vi "Waveform Acquisition - Process (4xI16).vi"(2 "Waveform Acquisition Resources":T1) -> ()   [LabVIEW 2018, in "Streaming FPGA.lvlib"]
doc: "Waveform Acquisition processing VI.\n\nConnect the <B>Waveform Acquisition Resources</B> input of this VI to the output of the <B>Waveform Acquisition - Create Resources.vi</B>."
uses:
  Streaming FPGA.lvlib
  Waveform Acquisition Resources (4xI16).ctl
  Target-Scoped FIFO (4xI16) Resource.ctl
  <vilib>/Platform/TimedLoop/XDataNode/timing_clust.ctl
  <vilib>/Platform/TimedLoop/XDataNode/nitl_modes.ctl
  <vilib>/Platform/TimedLoop/XDataNode/wakeup.ctl
  Data Storage - DRAM FIFO Priority.ctl
  <vilib>/rvi/Emulation/niFpgaSctlEmulationGetInTimedLoop.vi
  <vilib>/rvi/Emulation/niFpgaEmulationReportErrorSimple.vi
  <vilib>/rvi/Emulation/niFpgaGetClockAttributes.vi
  <vilib>/rvi/Emulation/niFpgaCriticalErrorInLSC.vi
  <vilib>/rvi/DataTransferAndStorage/Container/Common/niFpgaContainerExecOnDevCompGetState.vi
  <vilib>/rvi/Emulation/niFpgaEmulationIsFPGAContextNoSignature.vi
  <vilib>/rvi/DataTransferAndStorage/Container/Common/niFpgaContainerGetUniqueNameForEmu.vi
  <vilib>/rvi/Memory/Memory_Emulation/niFpgaMemoryEmulationCacheClearOnFirstRun.vi
  <vilib>/rvi/Memory/Memory_Emulation/nirvimemoryEmulationManagerCache_MakeExclusive.vi
  <vilib>/rvi/Memory/Memory_Emulation/niFpgaMemoryEmulationValidateCache.vi
  <vilib>/rvi/Memory/Memory_Emulation/nirvimemoryEmulationManagerCache_InsertValue.vi
  <vilib>/Utility/error.llb/Clear Errors.vi
  <vilib>/rvi/Memory/Memory_Emulation/nirvimemoryEmulationManagerCache_ReleaseExclusive.vi
  <vilib>/rvi/Memory/Memory_Emulation/nirvimemoryEmulationManagerCache_GetValue.vi
  <vilib>/rvi/Memory/Memory_Emulation/nirvimemoryEmulationManagerCache_SetValue.vi
  <vilib>/rvi/Emulation/niFpgaProcessEmulError.vi
  <instrlib>/_niInstr/Basic Elements/v1/FPGA/Private/Count Up U32.vi
  <vilib>/rvi/errors/niFpgaSetErrorForExecOnDevCompSimple.vi
  <vilib>/rvi/eio/common/nirviEmuReportErrorAndStop.vi
  <vilib>/rvi/interface/RandomDataEmulation/nirviRandomDataAcquireLock.vi
  <vilib>/rvi/interface/RandomDataEmulation/nirviRandomDataQueueStore.vi
  <vilib>/rvi/interface/RandomDataEmulation/nirviRandomDataReleaseLock.vi
  <vilib>/rvi/interface/RandomDataEmulation/nirviFPGAContextMergeError.vi
  <vilib>/rvi/interface/RandomDataEmulation/nirviRandomDataCheckExitLoopConditions.vi
  <vilib>/express/rvi/timingcommon/nirviCommon.vi
  <vilib>/rvi/interface/RandomDataEmulation/niFpgaRandomDataHandleErrors.vi
  <vilib>/platform/TimedLoop/XDataNode/XDataNode.xnode
  <vilib>/rvi/DataTransferAndStorage/Container/XNode/niFpgaContainer.xnode
  <vilib>/rvi/DataTransferAndStorage/Register/Emulation/niFpgaRegisterEmulationRefIn.vi
  <vilib>/rvi/FIFO/Fifo_Resource/niFpgaFifoEmulationRefInMultiElement.vi
  <vilib>/Platform/TimedLoop/XDataNode/XDNodeRunTimeDep.lvlib
  <instrlib>/_niInstr/Basic Elements/v1/FPGA/niInstr Basic Elements v1 FPGA.lvlib
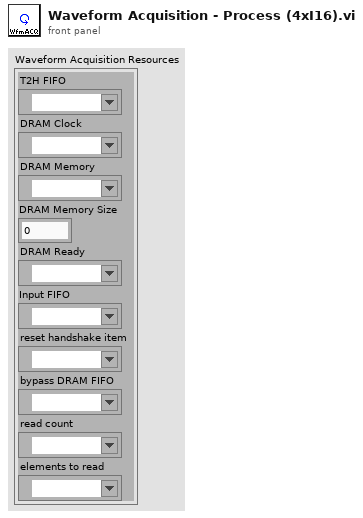
[diagram p1: front panel]
types:
  T1 = typedef "Streaming FPGA.lvlib/Waveform Acquisition Resources (4xI16).ctl" = cluster{"T2H FIFO":refnum<k21>, "DRAM Clock":refnum<k21>, "DRAM Memory":refnum<k21>, "DRAM Memory Size":u32, "DRAM Ready":refnum<k21>, "Input FIFO":T2, "reset handshake item":refnum<k21>, "bypass DRAM FIFO":refnum<k21>, "read count":refnum<k21>, "elements to read":refnum<k21>}
  T2 = typedef "Streaming FPGA.lvlib/Target-Scoped FIFO (4xI16) Resource.ctl" = refnum<k21>
  T3 = typedef "XDNodeRunTimeDep.lvlib/timing_clust.ctl" = cluster{"Expected End [f-1]":u64, "Actual End [f-1]":u64, "Finished Late? [f-1]":bool, "Expected End [i-1]":u64, "Actual End [i-1]":u64, "Finished Late? [i-1]":bool, "Expected Start [i]":u64, "Actual Start [i]":u64, "Expected Start [f]":u64, "Actual Start [f]":u64, "Source Name":string, "Structure Name":string, "Period":i64, "Deadline":i64, "Offset":i64, "Start":i64, "Priority":i32, "Timeout":i32, "Mode":T4, "Wakeup Reason":T5, "Error":errorcluster, "Source Type":string, "Secondary Source Type":string, "Global End Time":u64, "Global Start Time":u64, "Frame Duration":u64, "Iteration Duration":u64, "Assigned CPU":i32, "I/O Scan Engine Mode":u32}
  T4 = typedef "XDNodeRunTimeDep.lvlib/nitl_modes.ctl" = enum32{"No Change", "Process missed periods, maintain original phase", "Discard missed periods, maintain original phase", "Process missed periods, ignore original phase", "Discard missed periods, ignore original phase"}
  T5 = typedef "XDNodeRunTimeDep.lvlib/wakeup.ctl" = enum32{"Normal", "Aborted", "Asynchronous wakeup", "Timing source error", "Timed loop error", "Timeout"}
  T6 = typedef "Streaming FPGA.lvlib/Data Storage - DRAM FIFO Priority.ctl" = enum16{"balanced", "favor writes", "favor reads"}
  T7 = typedef "Streaming FPGA.lvlib/Data Type (4xI16).ctl" = i16[]
  T8 = typedef "Streaming FPGA.lvlib/Data Type (16xI16).ctl" = i16[]
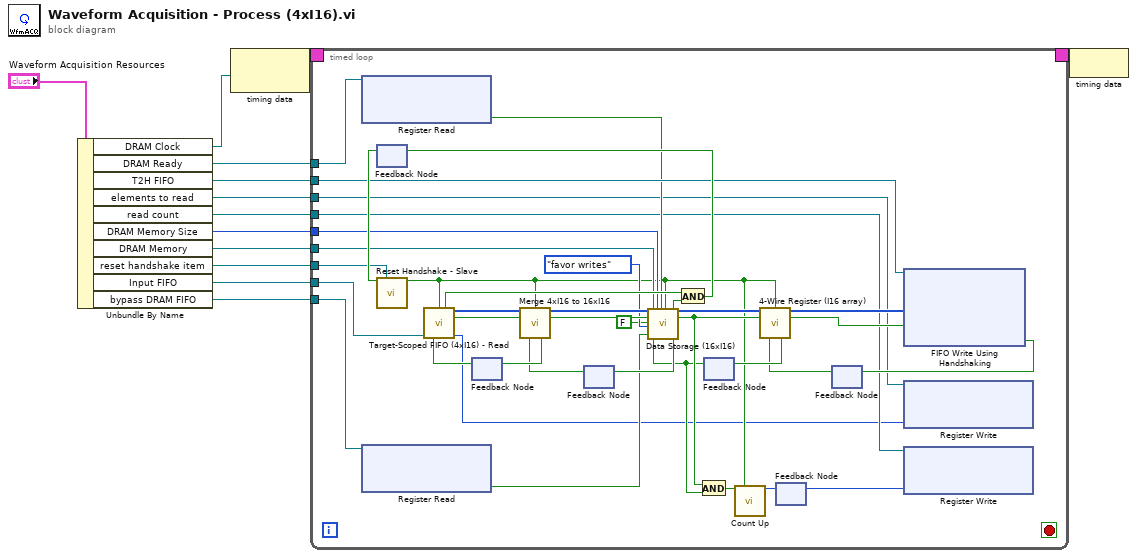
[diagram p0: block diagram]
diagram:
  n1 = Unbundle By Name("Waveform Acquisition Resources") -> ("DRAM Clock"=w7:refnum<k21>, "DRAM Ready"=w5:refnum<k21>, "T2H FIFO"=w6:refnum<k21>, "elements to read"=w2:refnum<k21>, "read count"=w1:refnum<k21>, "DRAM Memory Size"=w4:u32, "DRAM Memory"=w13:refnum<k21>, "reset handshake item"=w10:refnum<k21>, "Input FIFO"=w11:T2, "bypass DRAM FIFO"=w3:refnum<k21>)
  n2 = node-c288(w7) -> (w9:T3)
  n3 = timed-loop {
    timing: w9 -> [_]
    timing-out: [_] -> w8
    tunnel: w13 -> [w29]
    tunnel: w11 -> [w46]
    tunnel: w10 -> [w47]
    tunnel: w4 -> [w28]
    tunnel: w6 -> [w45]
    tunnel: w5 -> [w27]
    tunnel: w3 -> [w24]
    tunnel: w2 -> [w15]
    tunnel: w1 -> [w16]
    stop <- _ stop-if-true
    n4 = xnode "Register Read"("Register In"=w27) -> ("Data"=w26:bool)  [unwired: 1 out]
    n5 = xnode "Register Read"("Register In"=w24) -> ("Data"=w23:bool)  [unwired: 1 out]
    n6 = feedback #1() -> (w49:bool)  [unwired: 1 in]
    n7 = call "Reset Handshake - Slave.vi"("reset done"=w49, "reset handshake item"=w47) -> ("reset"=w19:bool)  [unwired: 13 in]
    n8 = feedback #2() -> (w40:bool)  [unwired: 1 in]
    n9 = call "Target-Scoped FIFO (4xI16) - Read.vi"("reset"=w19, "Target-Scoped FIFO (4xI16)"=w46, "ready for output (T)"=w40) -> ("reset done"=w50:bool, "data out"=w37:T7, "output valid"=w36:bool, "elements to read"=w14:u32)  [unwired: 9 in]
    n10 = feedback #3() -> (w32:bool)  [unwired: 1 in]
    n11 = call "Merge 4xI16 to 16xI16.vi"("data in"=w37, "reset"=w19, "input valid"=w36, "ready for output (T)"=w32) -> ("data out"=w34:i16[], "output valid"=w33:bool, "ready for input"=w35:bool)  [unwired: 9 in]
    n12 = feedback-in #2(w35) -> ()
    n13 = feedback #4() -> (w21:bool)  [unwired: 1 in]
    n14 = call "Data Storage (16xI16).vi"("data in"=w34, "input valid"=w33, "memory mode (F)"=FALSE, "priority (balanced)"=Data_Storage_-_DRAM_FIFO_Priority."favor writes", "bypass DRAM FIFO (F)"=w23, "DRAM Memory"=w29, "ready for output (T)"=w21, "Memory Size"=w28, "DRAM Ready"=w26, "reset"=w19) -> ("reset done"=w39:bool, "ready for input"=w31:bool, "data out"=w38:T8, "output valid"=w22:bool)  [unwired: 14 in]
    n15 = feedback-in #3(w31) -> ()
    n16 = And(x=w50, y=w39) -> (x .and. y?=w51:bool)
    n17 = feedback-in #1(w51) -> ()
    n18 = And(x=w22, y=w21) -> (x .and. y?=w20:bool)
    n19 = call-poly <instrlib>:"Count Up.vi"("increment"=w20, "reset"=w19) -> ("count out"=w18:u32)  [unwired: 13 in]
    n20 = feedback #5() -> (w17:u32)  [unwired: 1 in]
    n21 = feedback-in #5(w18) -> ()
    n22 = feedback #6() -> (w43:bool)  [unwired: 1 in]
    n23 = call "4-Wire Register (I16 array).vi"("data in"=w38, "reset"=w19, "input valid"=w22, "ready for output (T)"=w43) -> ("data out"=w42:i16[], "output valid"=w41:bool, "ready for input"=w48:bool)  [unwired: 9 in]
    n24 = feedback-in #4(w48) -> ()
    n25 = xnode "FIFO Write Using Handshaking"("Element"=w42, "Input Valid"=w41, "FIFO In"=w45) -> ("Ready for Input"=w44:bool)  [unwired: 1 out]
    n26 = feedback-in #6(w44) -> ()
    n27 = xnode "Register Write"("Data"=w14, "Register In"=w15) -> ()  [unwired: 1 out]
    n28 = xnode "Register Write"("Data"=w17, "Register In"=w16) -> ()  [unwired: 1 out]
  }
  n29 = node-c288(w8) -> ()
